vi "GetTrapSeparation(V).vi"(4 "ErrorIn":errorcluster, 5 "AcquisitionRatePerChannel":dbl, 7 "DAQ Task":refnum<k21>) -> (0 "ErrorOut":errorcluster, 1 "VertTrapSeparation(V)":dbl, 2 "HorTrapSeparation(V)":dbl, 3 "DAQ Task":refnum<k21>)   [LabVIEW 2012]
uses:
  <vilib>/DAQmx/configure/timing.llb/DAQmx Timing (Sample Clock).vi
  <vilib>/DAQmx/read.llb/DAQmx Read (Analog 2D DBL NChan NSamp).vi
  <vilib>/Analysis/baseanly.llb/Mean (DBL).vi
  <vilib>/Analysis/NI_AALBase.lvlib
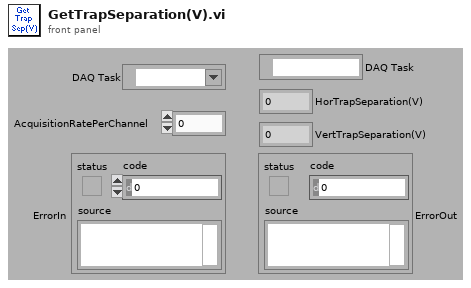
[diagram p1: front panel]
types:
  T1 = cluster{"[0]":dbl, "[1]":dbl, "[2]":dbl, "[3]":dbl, "[4]":dbl, "[5]":dbl, "[6]":dbl, "[7]":dbl}
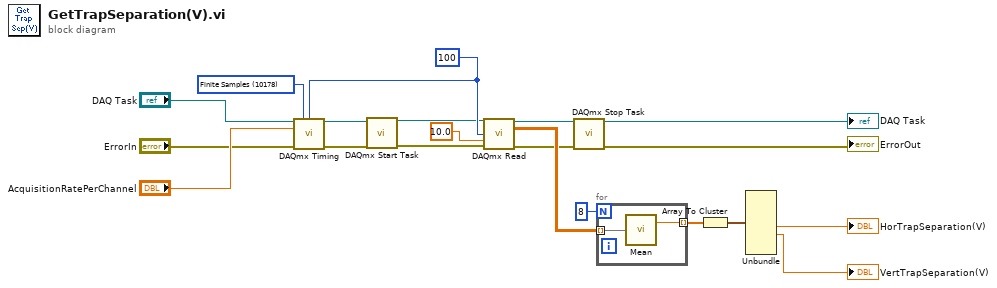
[diagram p0: block diagram]
diagram:
  w20 = 100 ("samples per channel")
  w4 = 10178 items=["Finite Samples"=10178, "Continuous Samples"=10123, "Hardware Timed Single Point"=12522] ("sample mode")
  n1 = call-poly <vilib>:"DAQmx Timing.vi"("task/channels in"="DAQ Task", "sample mode"=w4, "samples per channel"=w20, "rate"="AcquisitionRatePerChannel", "error in"="ErrorIn") -> ("task out"=w14:refnum<k21>, "error out"=w16:errorcluster)  [unwired: 9 in]
  n2 = call <vilib>:"DAQmx Start Task.vi"("task/channels in"=w14, "error in"=w16) -> ("task out"=w15:refnum<k21>, "error out"=w17:errorcluster)  [unwired: 12 in]
  n3 = call-poly <vilib>:"DAQmx Read.vi"("task/channels in"=w15, "number of samples per channel"=w20, "timeout"=10.0, "error in"=w17) -> ("task out"=w2:refnum<k21>, "data"=w11:dbl[][], "error out"=w3:errorcluster)  [unwired: 9 in]
  n4 = call <vilib>:"DAQmx Stop Task.vi"("task/channels in"=w2, "error in"=w3) -> ("task out"=→"DAQ Task":refnum<k21>, "error out"=→"ErrorOut":errorcluster)  [unwired: 12 in]
  n5 = for {
    N: 8 -> [_]
    tunnel: [w22] -> w10 mode=indexing
    tunnel: w11 -> [w21] mode=indexing
    n6 = call-poly <vilib>:"Mean.vi"("X"=w21) -> ("mean"=w22:dbl)  [unwired: 1 out]
  }
  n7 = Array To Cluster(array=w10) -> (cluster=w8:T1)
  n8 = Unbundle(w8) -> ("[4]"=→"HorTrapSeparation(V)":dbl, "[5]"=→"VertTrapSeparation(V)":dbl)  [unwired: 6 out]
